vi "Boiler.vi"() -> ()   [LabVIEW 2019]
uses:
  Controls/Sequence.ctl
panel:
  in  "Stop Button":bool
  out "error out":errorcluster
  in  "error in":errorcluster
  out "Status":T1
  in  "Boiler Simulation Controls":T2={"Fuel Control Valve Position (% Open)"=0.7016412776341991, "Flame Sensor Value (%)"=0.0, "Run Interlock"=FALSE, "Forced Draft Fan"=FALSE} {"Flame Sensor Value (%)" scale=0.0..100.0; "Fuel Control Valve Position (% Open)" scale=0.0..100.0}
  out "Boiler Status Indicators":T3 {"Time Counter(s)" format="%#.2f"}
  in  "Boiler Controls":T4
  # "Start/Stop"
  # "Fuel %"
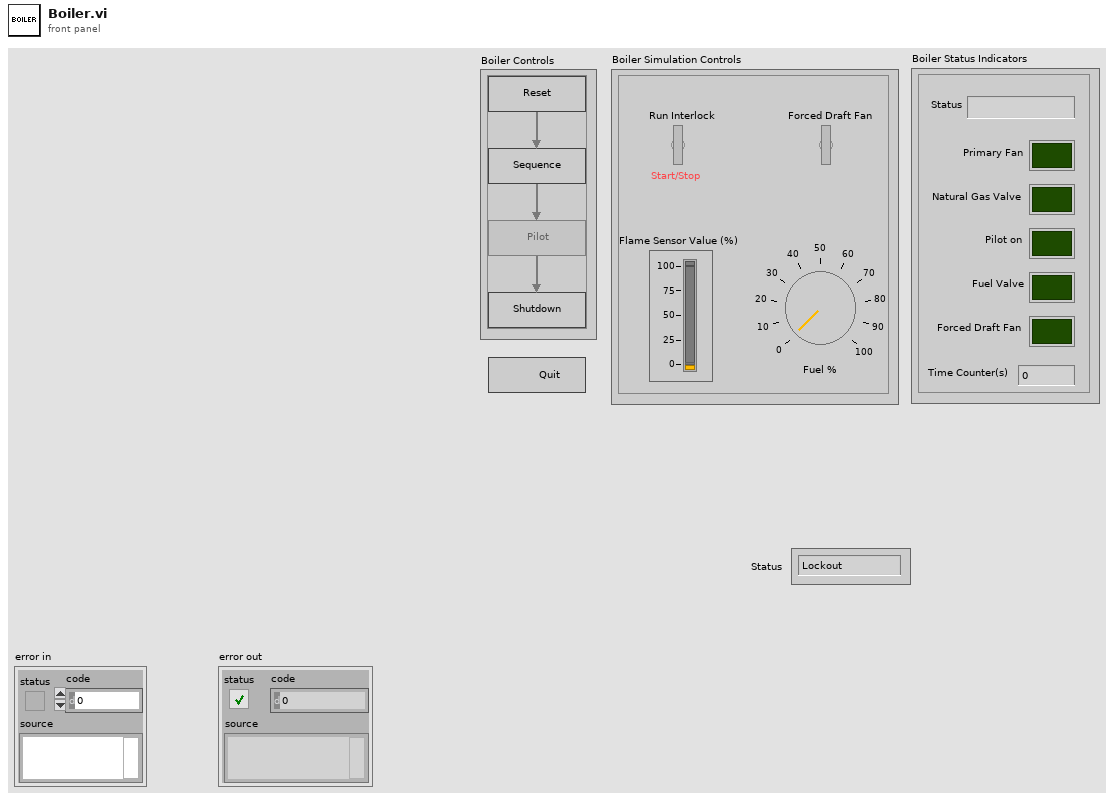
[diagram p1: front panel]
types:
  T1 = typedef "Sequence.ctl" = enum16{"Lockout", "Ready", "Pre-Purge", "Pilot On", "Boiler Ready", "Boiler Running", "Purge"}
  T2 = cluster{"Fuel Control Valve Position (% Open)":dbl, "Flame Sensor Value (%)":dbl, "Run Interlock":bool, "Forced Draft Fan":bool}
  T3 = cluster{"Primary Fan":bool, "Natural Gas Valve":bool, "Pilot on":bool, "Fuel Valve":bool, "Forced Draft Fan":bool, "Status":string, "Time Counter(s)":dbl}
  T4 = cluster{"Boiler Reset":bool, "Start Sequence":bool, "Pilot on":bool, "Shutdown":bool}
  T5 = enum8{"Enabled", "Disabled", "Disabled and Grayed Out"}
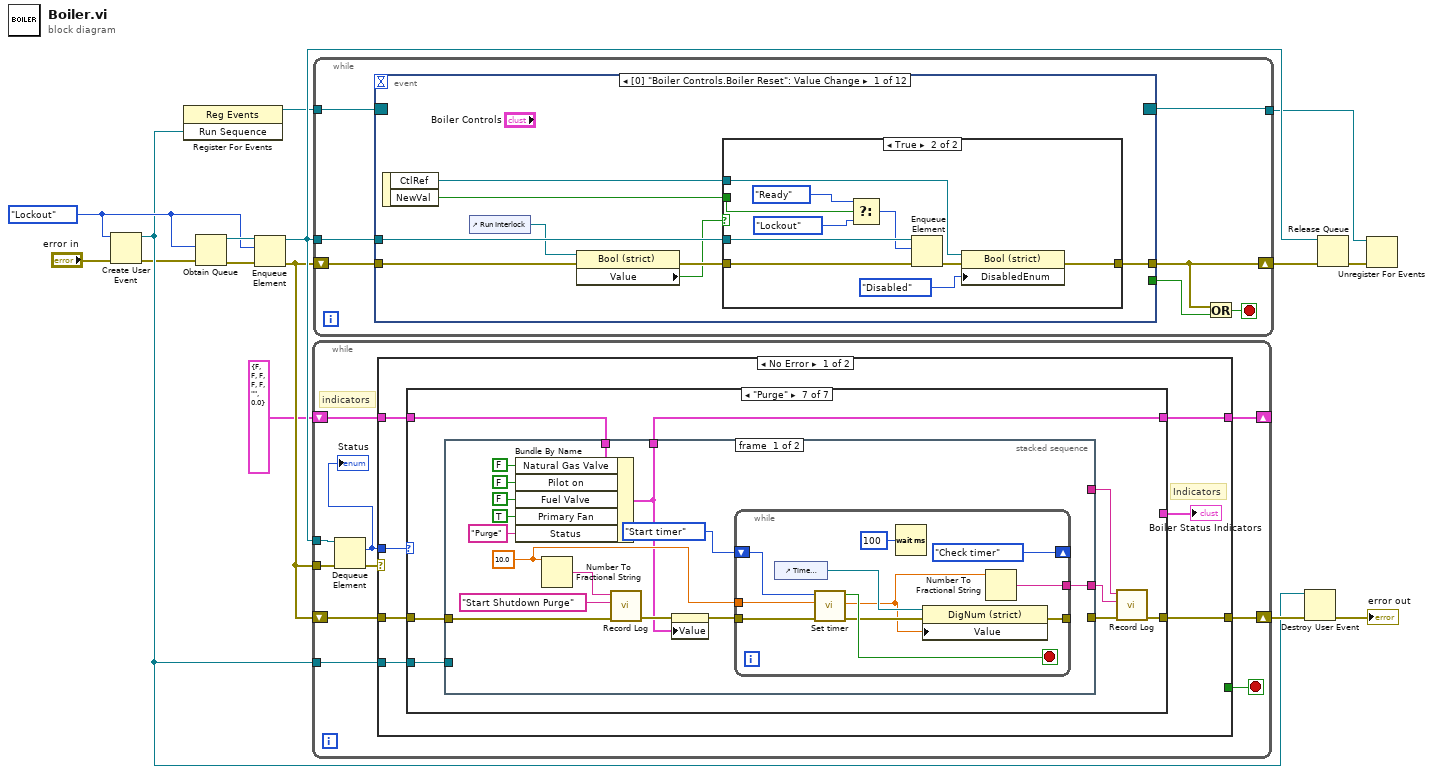
[diagram p0: block diagram]
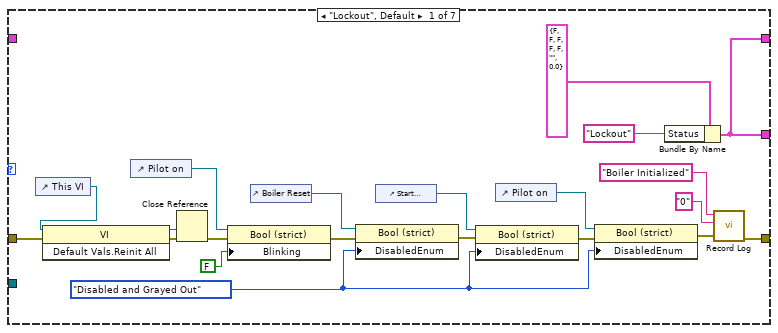
[diagram p2: hidden frame]
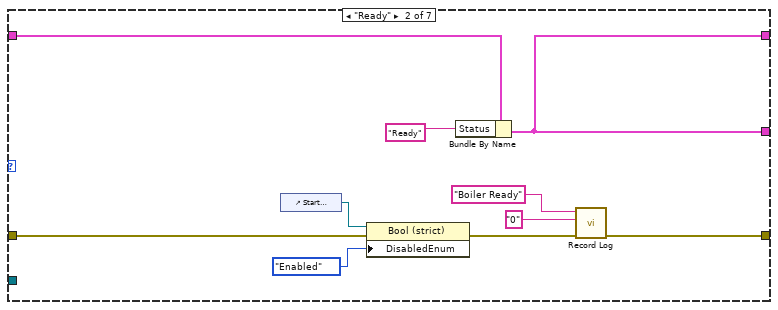
[diagram p3: hidden frame]
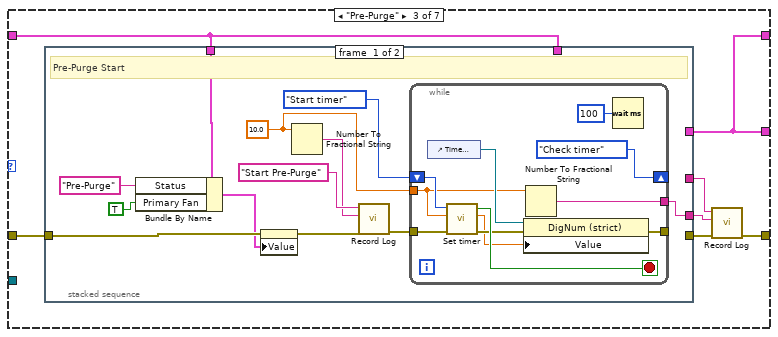
[diagram p4: hidden frame]
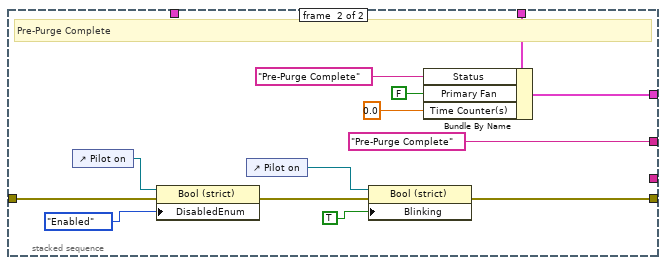
[diagram p5: hidden frame]
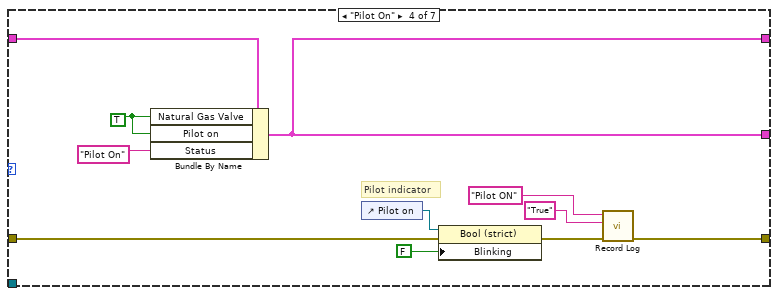
[diagram p6: hidden frame]
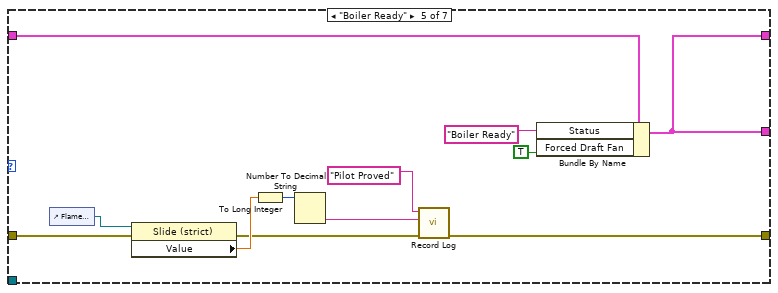
[diagram p7: hidden frame]
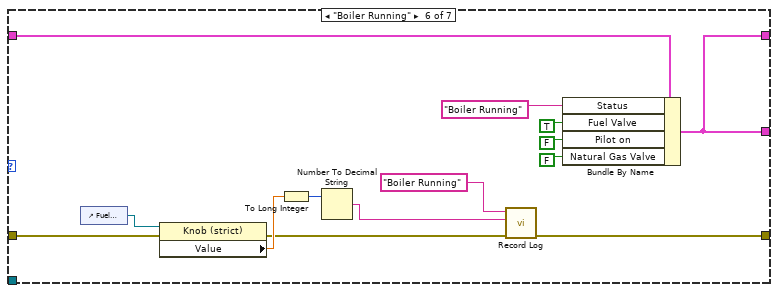
[diagram p8: hidden frame]
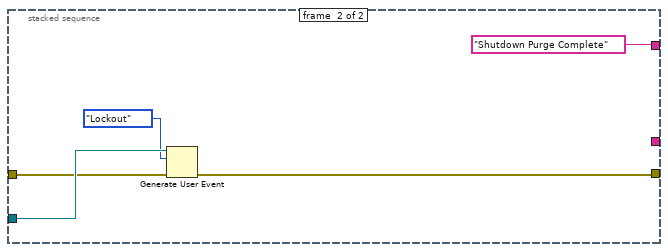
[diagram p9: hidden frame]
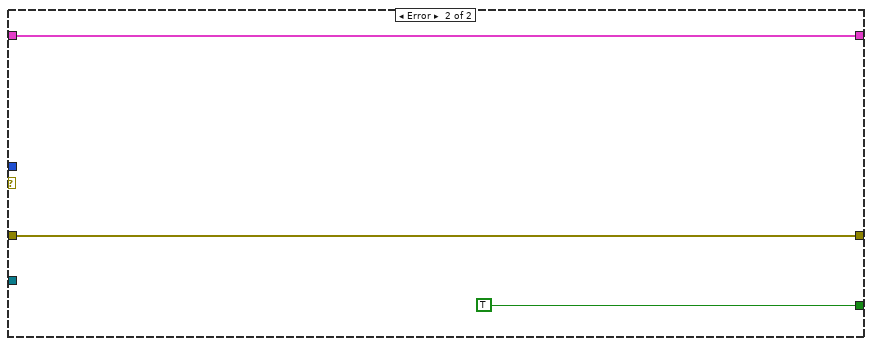
[diagram p10: hidden frame]
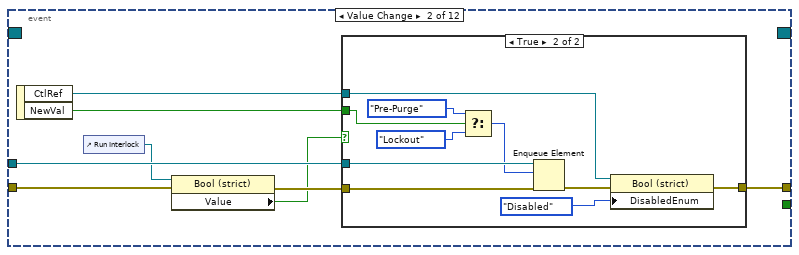
[diagram p12: hidden frame]
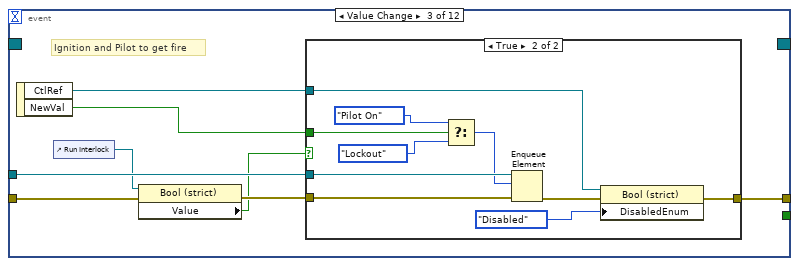
[diagram p14: hidden frame]
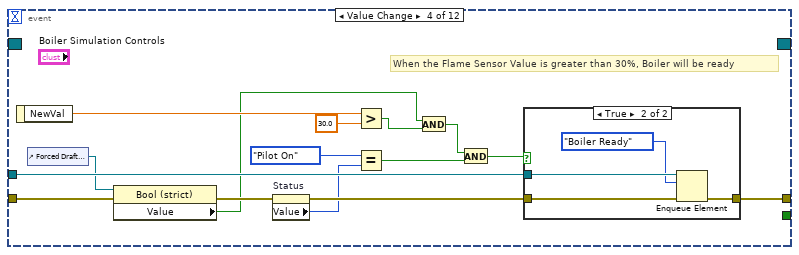
[diagram p16: hidden frame]
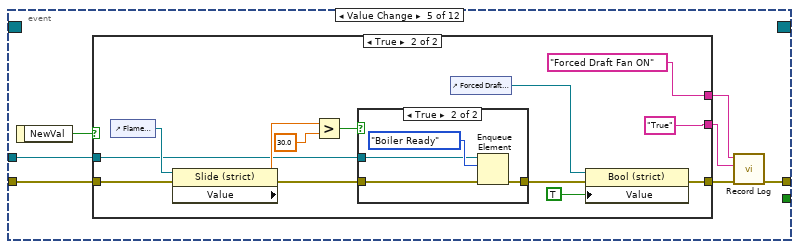
[diagram p18: hidden frame]
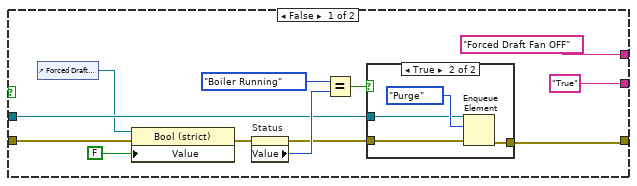
[diagram p19: hidden frame]
diagram:
  w9 = Sequence."Lockout" ("Run Sequence")
  n1 = Create User Event(user event datatype=w9, error in="error in") -> (user event=w5:refnum<user-event>, error out=w1:errorcluster)
  n2 = register-events(w5) -> (reference out=w8:refnum<event-registration>)  [unwired: 2 in, 1 out]
  n3 = Obtain Queue(element data type=w9, error in (no error)=w1) -> (queue out=w13:refnum<queue>, error out=w15:errorcluster)  [unwired: 3 in, 1 out]
  n4 = Enqueue Element(queue=w13, element=w9, error in (no error)=w15) -> (queue out=w14:refnum<queue>, error out=w12:errorcluster)  [unwired: 1 in, 1 out]
  n5 = while {
    shift-right: [w24] -> w7
    shift-left: w12 -> [w23]
    tunnel: w14 -> [w25]
    tunnel: w12 -> [w21]
    shift-right: [w19] -> _
    shift-left: T3 {"Primary Fan"=FALSE, "Natural Gas Valve"=FALSE, "Pilot on"=FALSE, "Fuel Valve"=FALSE, "Forced Draft Fan"=FALSE, "Status"="", "Time Counter(s)"=0.0} ("Boiler Status Indicators") -> [w18]
    tunnel: w5 -> [w16]
    stop <- w20 stop-if-true
    # "indicators"
    n6 = Dequeue Element(queue=w25, error in (no error)=w21) -> (element=w17:T1, error out=w22:errorcluster)  [unwired: 1 in, 2 out]
    "Status" <- w17
    n7 = case shown="No Error" w22 {
      tunnel: [w28 w185] -> w24
      tunnel: w17 -> [w31 _]
      tunnel: w23 -> [w32 w185]
      tunnel: [_ TRUE] -> w20
      tunnel: [w30 w183] -> w19
      tunnel: w18 -> [w29 w183]
      tunnel: w16 -> [w27 _]
      frame No Error {
        # "Indicators"
        n8 = case shown="\"Purge\"" w31 {
          tunnel: [w53 w60 w67 w117 w125 w134 w148] -> w28
          tunnel: w32 -> [w33 w55 w69 w107 w126 w135 w151]
          tunnel: [w41 w58 w66 w109 w119 w130 _] -> w26
          tunnel: [w41 w58 w66 w109 w119 w130 w149] -> w30
          tunnel: w29 -> [_ w59 w64 w108 w120 w136 w150]
          tunnel: w27 -> [_ _ _ _ _ _ w145]
          frame "Lockout", Default {
            w43 = T5."Disabled and Grayed Out" ("Disabled")
            n9 = control-ref of="This VI"() -> (w34:refnum<vi>)
            n10 = invoke class="VI" method="Default Vals.Reinit All"(reference=w34, error in=w33) -> (reference out=w36:refnum<vi>, error out=w37:errorcluster)  [unwired: 1 in, 1 out]
            n11 = control-ref of="Pilot on"() -> (w40:refnum<vi>)
            n12 = Close Reference(reference=w36, error in (no error)=w37) -> (error out=w35:errorcluster)
            n13 = property class="Bool (strict)"(reference=w40, error in=w35, "Blinking"=FALSE) -> (error out=w39:errorcluster)  [unwired: 1 out]
            n14 = control-ref of="Boiler Reset"() -> (w42:refnum<vi>)
            n15 = property class="Bool (strict)"(reference=w42, error in=w39, "DisabledEnum"=w43) -> (error out=w44:errorcluster)  [unwired: 1 out]
            n16 = control-ref of="Start Sequence"() -> (w46:refnum<vi>)
            n17 = property class="Bool (strict)"(reference=w46, error in=w44, "DisabledEnum"=w43) -> (error out=w48:errorcluster)  [unwired: 1 out]
            n18 = control-ref of="Pilot on"() -> (w45:refnum<vi>)
            n19 = property class="Bool (strict)"(reference=w45, error in=w48, "DisabledEnum"=w43) -> (error out=w47:errorcluster)  [unwired: 1 out]
            n20 = Bundle By Name(cluster=T3 {"Primary Fan"=FALSE, "Natural Gas Valve"=FALSE, "Pilot on"=FALSE, "Fuel Valve"=FALSE, "Forced Draft Fan"=FALSE, "Status"="", "Time Counter(s)"=0.0} ("Boiler Status Indicators"), "Status"="Lockout") -> (w41:T3)
            n21 = call "Record Log.vi"("Error In"=w47, "Data"="0" ("Data String"), "Event"="Boiler Initialized" ("Event String")) -> ("Error Out"=w53:errorcluster)  [unwired: 8 in]
          }
          frame "Ready" {
            n22 = control-ref of="Start Sequence"() -> (w57:refnum<vi>)
            n23 = property class="Bool (strict)"(reference=w57, error in=w55, "DisabledEnum"=T5."Enabled" ("Disabled")) -> (error out=w56:errorcluster)  [unwired: 1 out]
            n24 = Bundle By Name(cluster=w59, "Status"="Ready") -> (w58:T3)
            n25 = call "Record Log.vi"("Error In"=w56, "Data"="0" ("Data String"), "Event"="Boiler Ready" ("Event String")) -> ("Error Out"=w60:errorcluster)  [unwired: 8 in]
          }
          frame "Pre-Purge" {
            n26 = stacked-sequence {
              tunnel: [_ w100] -> w68
              tunnel: [_ w102] -> w66
              tunnel: [_ "Pre-Purge Complete" ("Event String")] -> w70
              tunnel: w69 -> [w72 w94]
              tunnel: w64 -> [w80 _]
              tunnel: [w74 _] -> w65
              tunnel: w64 -> [_ w99]
              frame #0 {
                w76 = 10.0 ("Time Target (s)")
                # "Pre-Purge Start"
                n27 = Bundle By Name(cluster=w80, "Status"="Pre-Purge" ("Event String"), "Primary Fan"=TRUE) -> (w71:T3)
                n28 = property on="Boiler Status Indicators" class="Clust (strict)"(error in=w72, "Value"=w71) -> (error out=w73:errorcluster)  [unwired: 1 in, 1 out]
                n29 = Number To Fractional String(number=w76) -> (F-format string=w78:string)  [unwired: 3 in]
                n30 = call "Record Log.vi"("Error In"=w73, "Data"=w78, "Event"="Start Pre-Purge" ("Event String")) -> ("Error Out"=w77:errorcluster)  [unwired: 8 in]
                n31 = while {
                  tunnel: w76 -> [w86]
                  tunnel: w77 -> [w93]
                  shift-right: [enum16{"Start timer", "Check timer"}."Check timer" ("Timer Commands")] -> _
                  shift-left: enum16{"Start timer", "Check timer"}."Start timer" ("Timer Commands") -> [w92]
                  tunnel: [w88] -> _
                  tunnel: [w85] -> w74
                  stop <- w91 stop-if-true
                  n32 = control-ref of="Time Counter(s)"() -> (w90:refnum<vi>)
                  n33 = call "Set timer.vi"("Error In"=w93, "Target Duration (s)"=w86, "Timer Commands"=w92) -> ("Error Out"=w89:errorcluster, "Elabsed Time(s)"=w87:dbl, "Done?"=w91:bool)  [unwired: 4 in]
                  n34 = property class="DigNum (strict)"(reference=w90, error in=w89, "Value"=w87) -> (error out=w88:errorcluster)  [unwired: 1 out]
                  n35 = Number To Fractional String(number=w86) -> (F-format string=w85:string)  [unwired: 3 in]
                  n36 = Wait (ms)(milliseconds to wait=u32 100) -> ()  [unwired: 1 out]
                }
              }
              frame #1 {
                # "Pre-Purge Complete"
                n37 = control-ref of="Pilot on"() -> (w97:refnum<vi>)
                n38 = property class="Bool (strict)"(reference=w97, error in=w94, "DisabledEnum"=T5."Enabled" ("Disabled")) -> (error out=w95:errorcluster)  [unwired: 1 out]
                n39 = control-ref of="Pilot on"() -> (w98:refnum<vi>)
                n40 = property class="Bool (strict)"(reference=w98, error in=w95, "Blinking"=TRUE) -> (error out=w100:errorcluster)  [unwired: 1 out]
                n41 = Bundle By Name(cluster=w99, "Status"="Pre-Purge Complete" ("Event String"), "Primary Fan"=FALSE, "Time Counter(s)"=0.0 ("Time Count (s)")) -> (w102:T3)
              }
            }
            n42 = call "Record Log.vi"("Error In"=w68, "Data"=w65, "Event"=w70) -> ("Error Out"=w67:errorcluster)  [unwired: 8 in]
          }
          frame "Pilot On" {
            w116 = TRUE ("Natural Gas Valve")
            # "Pilot indicator"
            n43 = Bundle By Name(cluster=w108, "Natural Gas Valve"=w116, "Pilot on"=w116, "Status"="Pilot On") -> (w109:T3)
            n44 = control-ref of="Pilot on"() -> (w113:refnum<vi>)
            n45 = property class="Bool (strict)"(reference=w113, error in=w107, "Blinking"=FALSE) -> (error out=w112:errorcluster)  [unwired: 1 out]
            n46 = call "Record Log.vi"("Error In"=w112, "Data"="True" ("Data String"), "Event"="Pilot ON" ("Event String")) -> ("Error Out"=w117:errorcluster)  [unwired: 8 in]
          }
          frame "Boiler Ready" {
            n47 = control-ref of="Flame Sensor Value (%)"() -> (w127:refnum<vi>)
            n48 = property class="Slide (strict)"(reference=w127, error in=w126) -> (error out=w124:errorcluster, "Value"=w129:dbl)  [unwired: 1 out]
            n49 = To Long Integer(number=w129) -> (32bit integer=w128:i32)
            n50 = Number To Decimal String(number=w128) -> (decimal integer string=w122:string)  [unwired: 1 in]
            n51 = call "Record Log.vi"("Error In"=w124, "Data"=w122, "Event"="Pilot Proved" ("Event String")) -> ("Error Out"=w125:errorcluster)  [unwired: 8 in]
            n52 = Bundle By Name(cluster=w120, "Status"="Boiler Ready", "Forced Draft Fan"=TRUE) -> (w119:T3)
          }
          frame "Boiler Running" {
            n53 = control-ref of="Fuel Control Valve Position (% Open)"() -> (w138:refnum<vi>)
            n54 = property class="Knob (strict)"(reference=w138, error in=w135) -> (error out=w133:errorcluster, "Value"=w139:dbl)  [unwired: 1 out]
            n55 = To Long Integer(number=w139) -> (32bit integer=w140:i32)
            n56 = Number To Decimal String(number=w140) -> (decimal integer string=w132:string)  [unwired: 1 in]
            n57 = call "Record Log.vi"("Error In"=w133, "Data"=w132, "Event"="Boiler Running" ("Event String")) -> ("Error Out"=w134:errorcluster)  [unwired: 8 in]
            n58 = Bundle By Name(cluster=w136, "Status"="Boiler Running", "Fuel Valve"=TRUE, "Pilot on"=FALSE ("Pilot Indicator"), "Natural Gas Valve"=FALSE) -> (w130:T3)
          }
          frame "Purge" {
            n59 = stacked-sequence {
              tunnel: [_ w179] -> w147
              tunnel: w151 -> [w161 w180]
              tunnel: w150 -> [w162 _]
              tunnel: [w154 _] -> w149
              tunnel: [w157 _] -> w146
              tunnel: w145 -> [_ w182]
              tunnel: [_ "Shutdown Purge Complete" ("Event String")] -> w144
              frame #0 {
                w158 = 10.0 ("Time Target (s)")
                n60 = Bundle By Name(cluster=w162, "Natural Gas Valve"=FALSE, "Pilot on"=FALSE, "Fuel Valve"=FALSE, "Primary Fan"=TRUE, "Status"="Purge") -> (w154:T3)
                n61 = Number To Fractional String(number=w158) -> (F-format string=w160:string)  [unwired: 3 in]
                n62 = call "Record Log.vi"("Error In"=w161, "Data"="Start Shutdown Purge" ("Event String"), "Event"=w160) -> ("Error Out"=w155:errorcluster)  [unwired: 8 in]
                n63 = property on="Boiler Status Indicators" class="Clust (strict)"(error in=w155, "Value"=w154) -> (error out=w156:errorcluster)  [unwired: 1 in, 1 out]
                n64 = while {
                  tunnel: w158 -> [w176]
                  tunnel: w156 -> [w177]
                  shift-right: [enum16{"Start timer", "Check timer"}."Check timer" ("Timer Commands")] -> _
                  shift-left: enum16{"Start timer", "Check timer"}."Start timer" ("Timer Commands") -> [w175]
                  tunnel: [w170] -> _
                  tunnel: [w167] -> w157
                  stop <- w173 stop-if-true
                  n65 = control-ref of="Time Counter(s)"() -> (w172:refnum<vi>)
                  n66 = call "Set timer.vi"("Error In"=w177, "Target Duration (s)"=w176, "Timer Commands"=w175) -> ("Error Out"=w171:errorcluster, "Elabsed Time(s)"=w168:dbl, "Done?"=w173:bool)  [unwired: 4 in]
                  n67 = Wait (ms)(milliseconds to wait=u32 100) -> ()  [unwired: 1 out]
                  n68 = property class="DigNum (strict)"(reference=w172, error in=w171, "Value"=w168) -> (error out=w170:errorcluster)  [unwired: 1 out]
                  n69 = Number To Fractional String(number=w168) -> (F-format string=w167:string)  [unwired: 3 in]
                }
              }
              frame #1 {
                n70 = Generate User Event(user event=w182, event data cluster=Sequence."Lockout" ("event data"), error in=w180) -> (error out=w179:errorcluster)  [unwired: 1 in, 1 out]
              }
            }
            n71 = call "Record Log.vi"("Error In"=w147, "Data"=w146, "Event"=w144) -> ("Error Out"=w148:errorcluster)  [unwired: 8 in]
          }
        }
        "Boiler Status Indicators" <- w26
      }
      frame Error {
      }
    }
  }
  n72 = while {
    shift-right: [w189] -> w4
    shift-left: w12 -> [w188]
    tunnel: w14 -> [w192]
    tunnel: w8 -> [w187]
    tunnel: [w186] -> w10
    stop <- w191 stop-if-true
    n73 = event shown="[0] \"Boiler Controls.Boiler Reset\": Value Change" {
      selector: w187 -> [_ _ _ _ _ _ _ _ _ _ _ _]
      dyn-events: [_ _ _ _ _ _ _ _ _ _ _ _] -> w186
      timeout: _ -> [_ _ _ _ _ _ _ _ _ _ _ _]
      tunnel: w192 -> [w199 w219 w238 w264 w272 w325 w341 w350 w382 _ w410 _]
      tunnel: w188 -> [w196 w216 w235 w256 w270 w314 w337 w351 w383 w408 w412 w414]
      tunnel: [w200 w218 w237 w263 w276 w326 w342 w349 w381 w408 w411 w414] -> w189
      tunnel: [_ _ _ _ _ _ _ _ _ w407 _ TRUE ("NewVal")] -> w190
      event "Boiler Controls.Boiler Reset": Value Change {
        n74 = event-data() -> ("CtlRef"=w193:refnum<vi>, "NewVal"=w198:bool)  [unwired: 1 in]
        n75 = control-ref of="Run Interlock"() -> (w197:refnum<vi>)
        n76 = property class="Bool (strict)"(reference=w197, error in=w196) -> (error out=w195:errorcluster, "Value"=w194:bool)  [unwired: 1 out]
        n77 = case shown="True" w194 {
          tunnel: [w201 w203] -> w200
          tunnel: w199 -> [_ w211]
          tunnel: w198 -> [_ w207]
          tunnel: w195 -> [w201 w206]
          tunnel: w193 -> [_ w202]
          frame False {
          }
          frame True {
            n78 = Select(t=Sequence."Ready" ("Set Function"), s=w207, f=Sequence."Lockout" ("Set Function")) -> (s? t:f=w208:T1)
            n79 = Enqueue Element(queue=w211, element=w208, error in (no error)=w206) -> (error out=w204:errorcluster)  [unwired: 1 in, 2 out]
            n80 = property class="Bool (strict)"(reference=w202, error in=w204, "DisabledEnum"=T5."Disabled" ("Disabled")) -> (error out=w203:errorcluster)  [unwired: 1 out]
          }
        }
      }
      event "Boiler Controls.Start Sequence": Value Change {
        n81 = event-data() -> ("CtlRef"=w212:refnum<vi>, "NewVal"=w213:bool)  [unwired: 1 in]
        n82 = control-ref of="Run Interlock"() -> (w217:refnum<vi>)
        n83 = property class="Bool (strict)"(reference=w217, error in=w216) -> (error out=w215:errorcluster, "Value"=w214:bool)  [unwired: 1 out]
        n84 = case shown="True" w214 {
          tunnel: w219 -> [_ w230]
          tunnel: [w220 w223] -> w218
          tunnel: w213 -> [_ w226]
          tunnel: w215 -> [w220 w225]
          tunnel: w212 -> [_ w222]
          frame False {
          }
          frame True {
            n85 = Select(t=Sequence."Pre-Purge" ("Run Sequence"), s=w226, f=Sequence."Lockout" ("Run Sequence")) -> (s? t:f=w227:T1)
            n86 = Enqueue Element(queue=w230, element=w227, error in (no error)=w225) -> (error out=w224:errorcluster)  [unwired: 1 in, 2 out]
            n87 = property class="Bool (strict)"(reference=w222, error in=w224, "DisabledEnum"=T5."Disabled" ("Disabled")) -> (error out=w223:errorcluster)  [unwired: 1 out]
          }
        }
      }
      event "Boiler Controls.Pilot on": Value Change {
        # "Ignition and Pilot to get fire"
        n88 = event-data() -> ("CtlRef"=w231:refnum<vi>, "NewVal"=w232:bool)  [unwired: 1 in]
        n89 = control-ref of="Run Interlock"() -> (w236:refnum<vi>)
        n90 = property class="Bool (strict)"(reference=w236, error in=w235) -> (error out=w234:errorcluster, "Value"=w233:bool)  [unwired: 1 out]
        n91 = case shown="True" w233 {
          tunnel: w238 -> [_ w249]
          tunnel: [w239 w241] -> w237
          tunnel: w234 -> [w239 w248]
          tunnel: w232 -> [_ w247]
          tunnel: w231 -> [_ w240]
          frame False {
          }
          frame True {
            n92 = Select(t=Sequence."Pilot On" ("Run Sequence"), s=w247, f=Sequence."Lockout" ("Run Sequence")) -> (s? t:f=w244:T1)
            n93 = Enqueue Element(queue=w249, element=w244, error in (no error)=w248) -> (error out=w242:errorcluster)  [unwired: 1 in, 2 out]
            n94 = property class="Bool (strict)"(reference=w240, error in=w242, "DisabledEnum"=T5."Disabled" ("Disabled")) -> (error out=w241:errorcluster)  [unwired: 1 out]
          }
        }
      }
      event "Boiler Simulation Controls.Flame Sensor Value (%)": Value Change {
        # "When the Flame Sensor Value is greater than 30%, Boiler will be ready"
        n95 = event-data() -> ("NewVal"=w261:dbl)  [unwired: 1 in]
        n96 = control-ref of="Forced Draft Fan"() -> (w257:refnum<vi>)
        n97 = property class="Bool (strict)"(reference=w257, error in=w256) -> (error out=w255:errorcluster, "Value"=w253:bool)  [unwired: 1 out]
        n98 = property on="Status" class="Enum (strict)"(error in=w255) -> (error out=w260:errorcluster, "Value"=w258:T1)  [unwired: 1 in, 1 out]
        n99 = Greater?(x=w261, y=30.0) -> (0:w254:bool)
        n100 = Equal?(x=Sequence."Pilot On" ("Run Sequence"), y=w258) -> (x = y?=w252:bool)
        n101 = And(x=w253, y=w254) -> (x .and. y?=w251:bool)
        n102 = And(x=w251, y=w252) -> (x .and. y?=w250:bool)
        n103 = case shown="True" w250 {
          tunnel: w264 -> [_ w269]
          tunnel: [w265 w268] -> w263
          tunnel: w260 -> [w265 w266]
          frame False {
          }
          frame True {
            n104 = Enqueue Element(queue=w269, element=Sequence."Boiler Ready" ("Run Sequence"), error in (no error)=w266) -> (error out=w268:errorcluster)  [unwired: 1 in, 2 out]
          }
        }
      }
      event "Boiler Simulation Controls.Forced Draft Fan": Value Change {
        n105 = event-data() -> ("NewVal"=w271:bool)  [unwired: 1 in]
        n106 = case shown="True" w271 {
          tunnel: [w282 w303] -> w275
          tunnel: ["Forced Draft Fan OFF" ("Event") "Forced Draft Fan ON" ("Event")] -> w273
          tunnel: ["True" ("Data") "True" ("Data")] -> w274
          tunnel: w272 -> [w281 w295]
          tunnel: w270 -> [w277 w300]
          frame False {
            n107 = control-ref of="Forced Draft Fan"() -> (w280:refnum<vi>)
            n108 = property class="Bool (strict)"(reference=w280, error in=w277, "Value"=FALSE) -> (error out=w278:errorcluster)  [unwired: 1 out]
            n109 = property on="Status" class="Enum (strict)"(error in=w278) -> (error out=w283:errorcluster, "Value"=w286:T1)  [unwired: 1 in, 1 out]
            n110 = Equal?(x=Sequence."Boiler Running" ("Run Sequence"), y=w286) -> (x = y?=w284:bool)
            n111 = case shown="True" w284 {
              tunnel: w283 -> [w289 w292]
              tunnel: [w289 w291] -> w282
              tunnel: w281 -> [_ w290]
              frame False {
              }
              frame True {
                n112 = Enqueue Element(queue=w290, element=Sequence."Purge" ("Run Sequence"), error in (no error)=w292) -> (error out=w291:errorcluster)  [unwired: 1 in, 2 out]
              }
            }
          }
          frame True {
            n113 = control-ref of="Flame Sensor Value (%)"() -> (w301:refnum<vi>)
            n114 = property class="Slide (strict)"(reference=w301, error in=w300) -> (error out=w296:errorcluster, "Value"=w298:dbl)  [unwired: 1 out]
            n115 = Greater?(x=w298, y=30.0) -> (0:w294:bool)
            n116 = case shown="True" w294 {
              tunnel: w296 -> [w307 w310]
              tunnel: [w307 w309] -> w297
              tunnel: w295 -> [_ w308]
              frame False {
              }
              frame True {
                n117 = Enqueue Element(queue=w308, element=Sequence."Boiler Ready" ("Run Sequence"), error in (no error)=w310) -> (error out=w309:errorcluster)  [unwired: 1 in, 2 out]
              }
            }
            n118 = control-ref of="Forced Draft Fan"() -> (w302:refnum<vi>)
            n119 = property class="Bool (strict)"(reference=w302, error in=w297, "Value"=TRUE) -> (error out=w303:errorcluster)  [unwired: 1 out]
          }
        }
        n120 = call "Record Log.vi"("Error In"=w275, "Data"=w274, "Event"=w273) -> ("Error Out"=w276:errorcluster)  [unwired: 8 in]
      }
      event "Boiler Simulation Controls.Fuel Control Valve Position (% Open)": Mouse Up {
        # "Shutdown : Fuel Valve <10 or Fuel Valve >75 after running"
        n121 = event-data() -> ()  [unwired: 1 in, 1 out]
        n122 = control-ref of="Fuel Control Valve Position (% Open)"() -> (w315:refnum<vi>)
        n123 = property class="Knob (strict)"(reference=w315, error in=w314) -> (error out=w313:errorcluster, "Value"=w312:dbl)  [unwired: 1 out]
        n124 = property on="Status" class="Enum (strict)"(error in=w313) -> (error out=w321:errorcluster, "Value"=w323:T1)  [unwired: 1 in, 1 out]
        n125 = In Range and Coerce(upper limit=75.0 ("y"), x=w312, lower limit=10.0 ("y")) -> (In Range?=w317:bool)  [unwired: 1 out]
        n126 = Equal?(x=Sequence."Boiler Running" ("Run Sequence"), y=w323) -> (x = y?=w320:bool)
        n127 = Not(x=w317) -> (.not. x?=w316:bool)
        n128 = And(x=w316, y=w320) -> (x .and. y?=w324:bool)
        n129 = case shown="True" w324 {
          tunnel: [w327 w330] -> w326
          tunnel: w325 -> [_ w329]
          tunnel: w321 -> [w327 w328]
          frame False {
          }
          frame True {
            n130 = Enqueue Element(queue=w329, element=Sequence."Purge" ("Run Sequence"), error in (no error)=w328) -> (error out=w330:errorcluster)  [unwired: 1 in, 2 out]
          }
        }
      }
      event "Boiler Simulation Controls.Fuel Control Valve Position (% Open)": Value Change {
        n131 = event-data() -> ("NewVal"=w339:dbl)  [unwired: 1 in]
        n132 = property on="Status" class="Enum (strict)"(error in=w337) -> (error out=w336:errorcluster, "Value"=w335:T1)  [unwired: 1 in, 1 out]
        n133 = Greater?(x=w339, y=10.0) -> (0:w334:bool)
        n134 = Equal?(x=Sequence."Boiler Ready" ("Run Sequence"), y=w335) -> (x = y?=w333:bool)
        n135 = And(x=w334, y=w333) -> (x .and. y?=w332:bool)
        n136 = case shown="True" w332 {
          tunnel: [w343 w347] -> w342
          tunnel: w341 -> [_ w345]
          tunnel: w336 -> [w343 w344]
          frame False {
          }
          frame True {
            n137 = Enqueue Element(queue=w345, element=Sequence."Boiler Running" ("Run Sequence"), error in (no error)=w344) -> (error out=w347:errorcluster)  [unwired: 1 in, 2 out]
          }
        }
      }
      event "Boiler Controls.Shutdown": Value Change {
        n138 = event-data() -> ("NewVal"=w348:bool)  [unwired: 1 in]
        n139 = case shown="True" w348 {
          tunnel: w351 -> [w352 w357]
          tunnel: w350 -> [_ w354]
          tunnel: [w352 w353] -> w349
          frame False {
          }
          frame True {
            n140 = property on="Status" class="Enum (strict)"(error in=w357) -> (error out=w355:errorcluster, "Value"=w356:T1)  [unwired: 1 in, 1 out]
            n141 = case shown="\"Pilot On\"" w356 {
              tunnel: [w360 w362 w367 w371 w376 w378 w379] -> w353
              tunnel: w355 -> [w361 w364 w369 w372 w377 w378 w379]
              tunnel: w354 -> [w358 w363 w368 w373 w374 _ _]
              frame "Ready" {
                n142 = Enqueue Element(queue=w358, element=Sequence."Lockout" ("Run Sequence"), error in (no error)=w361) -> (error out=w360:errorcluster)  [unwired: 1 in, 2 out]
              }
              frame "Pre-Purge" {
                n143 = Enqueue Element(queue=w363, element=Sequence."Lockout" ("Run Sequence"), error in (no error)=w364) -> (error out=w362:errorcluster)  [unwired: 1 in, 2 out]
              }
              frame "Pilot On" {
                n144 = Enqueue Element(queue=w368, element=Sequence."Purge" ("Run Sequence"), error in (no error)=w369) -> (error out=w367:errorcluster)  [unwired: 1 in, 2 out]
              }
              frame "Boiler Ready" {
                n145 = Enqueue Element(queue=w373, element=Sequence."Purge" ("Run Sequence"), error in (no error)=w372) -> (error out=w371:errorcluster)  [unwired: 1 in, 2 out]
              }
              frame "Boiler Running" {
                n146 = Enqueue Element(queue=w374, element=Sequence."Purge" ("Run Sequence"), error in (no error)=w377) -> (error out=w376:errorcluster)  [unwired: 1 in, 2 out]
              }
              frame "Purge" {
              }
              frame "Lockout" {
              }
            }
          }
        }
      }
      event "Boiler Simulation Controls.Run Interlock": Value Change {
        n147 = event-data() -> ("NewVal"=w380:bool)  [unwired: 1 in]
        n148 = case shown="False" w380 {
          tunnel: w383 -> [w388 w405]
          tunnel: w382 -> [w387 _]
          tunnel: [w384 w403] -> w381
          frame False {
            n149 = Two Button Dialog(message="Stop?") -> (T button?=w385:bool)  [unwired: 2 in]
            n150 = case shown="True" w385 {
              tunnel: w388 -> [w389 w400]
              tunnel: w387 -> [_ w398]
              tunnel: [w390 w393] -> w384
              frame False {
                n151 = control-ref of="Run Interlock"() -> (w392:refnum<vi>)
                n152 = property class="Bool (strict)"(reference=w392, error in=w389, "Value"=TRUE) -> (error out=w390:errorcluster)  [unwired: 1 out]
              }
              frame True {
                n153 = property on="Status" class="Enum (strict)"(error in=w400) -> (error out=w399:errorcluster, "Value"=w402:T1)  [unwired: 1 in, 1 out]
                n154 = Equal?(x=Sequence."Boiler Running", y=w402) -> (x = y?=w397:bool)
                n155 = Select(t=Sequence."Purge" ("Run Sequence"), s=w397, f=Sequence."Lockout" ("Run Sequence")) -> (s? t:f=w396:T1)
                n156 = Enqueue Element(queue=w398, element=w396, error in (no error)=w399) -> (error out=w393:errorcluster)  [unwired: 1 in, 2 out]
              }
            }
          }
          frame True {
            n157 = control-ref of="Boiler Reset"() -> (w406:refnum<vi>)
            n158 = property class="Bool (strict)"(reference=w406, error in=w405, "DisabledEnum"=T5."Enabled" ("Disabled")) -> (error out=w403:errorcluster)  [unwired: 1 out]
          }
        }
      }
      event "Stop Button": Value Change {
        n159 = event-data() -> ("NewVal"=w407:bool)  [unwired: 1 in]
      }
      event User Event {
        n160 = event-data() -> ("Run Sequence"=w409:T1)  [unwired: 1 in, 4 out]
        n161 = Enqueue Element(queue=w410, element=w409, error in (no error)=w412) -> (error out=w411:errorcluster)  [unwired: 1 in, 2 out]
      }
      event Timeout {
        n162 = event-data() -> ()  [unwired: 1 in, 3 out]
      }
    }
    n163 = Or(x=w189, y=w190) -> (x .or. y?=w191:bool)
  }
  n164 = Destroy User Event(user event=w5, error in=w7) -> (error out=→"error out":errorcluster)
  n165 = Release Queue(queue=w14, error in (no error)=w4) -> (error out=w3:errorcluster)  [unwired: 1 in, 2 out]
  n166 = Unregister For Events(event registration refnum=w10, error in=w3) -> ()  [unwired: 1 out]
